vi "Configure External ALC.vi"(8 "error in (no error)":errorcluster, 9 "Enable External ALC Hold (F: Disable)":bool, 10 "External ALC Hold Source (0: Trigger1)":i32(ring) items=["Trigger1", "Trigger2 ", "Pulse"], 11 "VISA resource name":refnum<visa-resource-name>) -> (0 "error out":errorcluster, 3 "VISA resource name out":refnum<visa-resource-name>)   [LabVIEW 2018, in "Agilent PSG MXG Series.lvlib"]
doc: "Configure External ALC Hold settings.\n\n<B>Notes:</B>\n(1) This VI is valid only in N5171B, N5172B, N5181B, N5182B,, N5173B, N5183B."
uses:
  Agilent PSG MXG Series.lvlib
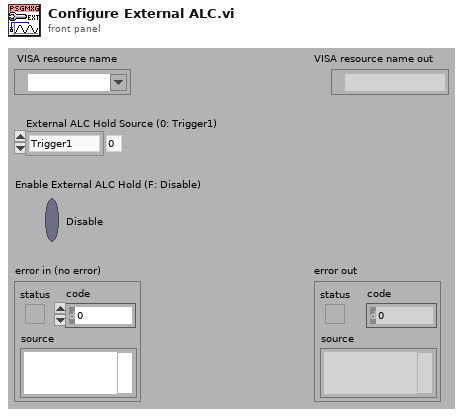
[diagram p1: front panel]
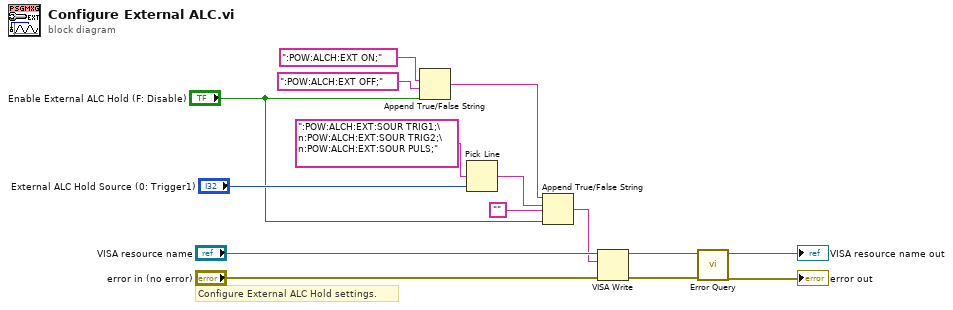
[diagram p0: block diagram]
diagram:
  # "Configure External ALC Hold settings."
  n1 = Append True/False String(1:"Enable External ALC Hold (F: Disable)", 2:":POW:ALCH:EXT OFF;", 3:":POW:ALCH:EXT ON;") -> (0:w4:string)  [unwired: 1 out]
  n2 = Pick Line(multi-line string=":POW:ALCH:EXT:SOUR TRIG1;\n:POW:ALCH:EXT:SOUR TRIG2;\n:POW:ALCH:EXT:SOUR PULS;", line index="External ALC Hold Source (0: Trigger1)") -> (output string=w3:string)  [unwired: 1 out]
  n3 = Append True/False String(1:"Enable External ALC Hold (F: Disable)", 2:"", 3:w3, 4:w4) -> (0:w1:string)
  n4 = VISA Write(VISA resource name="VISA resource name", write buffer=w1, error in (no error)="error in (no error)") -> (VISA resource name out=w9:refnum<visa-resource-name>, error out=w8:errorcluster)  [unwired: 1 out]
  n5 = call "Error Query.vi"("error in (no error)"=w8, "VISA resource name"=w9) -> ("error out"=→"error out":errorcluster, "VISA resource name out"=→"VISA resource name out":refnum<visa-resource-name>)  [unwired: 8 out]
